vi "COMI US Check File Convert.vi"() -> (3 "function return":sgl)   [LabVIEW 2017, in "Comidll.lvlib"]
doc: "float (COMI_US_CheckFileConvert) (void);"
uses:
  <userlib>/Comidll/Comidll.lvlib
  <userlib>/Comidll/Comidll.dll
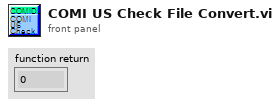
[diagram p1: front panel]
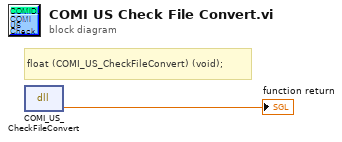
[diagram p0: block diagram]
diagram:
  # "float\t(COMI_US_CheckFileConvert) (void);"
  n1 = dll-call lib="C:/Program Files/National Instruments/LabVIEW 2017/user.lib/Comidll/Comidll.*" fn="COMI_US_CheckFileConvert"() -> (→"function return":sgl)  [unwired: 3 in, 2 out]
